vi "Pump Close Selection.vi"(8 "error in (no error)":errorcluster, 11 "Pump Settings In":T1 {"Masterflex"."Pump Number" min=1.0 max=20.0 step=1.0; "Ismatech"."Pump Number" min=1.0 max=20.0 step=1.0; "ASIA Pump C"."channel" min=-1 max=1 step=1}) -> (0 "error out":errorcluster, 1 "Connection Error":bool, 3 "Pump Settings Out":T1 {"Masterflex"."Pump Number" min=1.0 max=20.0 step=1.0; "Ismatech"."Pump Number" min=1.0 max=20.0 step=1.0; "ASIA Pump C"."channel" min=-1 max=1 step=1})   [LabVIEW 2018, in "Pump Module.lvlib" / "Pump Module Engine.lvlib"]
uses:
  Measure Instrument/Pump Module Engine.lvlib
  Measure Instrument/Pump Settings Cluster.ctl
  Measure Instrument/PID 2 Output Enum.ctl
  Masterflex 7550-30/Controls/Settings Cluster.ctl
  Ismatec ISM 831C/Controls/Ismatech Settings Cluster.ctl
  VICI M50 Party Mode/Settings Cluster.ctl
  Tacmina QI/Tacmina QI DAQ Setting.ctl
  KNF Pump/Settings Cluster plus SIMDOS.ctl
  ASIA Pump/Pump Settings.ctl
  FLOM Pump/Settings Cluster.ctl
  SSI PR Class/SSI PR Settings Cluster.ctl
  Ismatec ISM 831C/Ismatec ISM 831C.lvlib
  Masterflex 7550-30/Masterflex 7550-30.lvlib
  VICI M50 Party Mode/VICI M6 M50 Party Mode.lvlib
  Tacmina QI/Tacmina QI.lvlib
  KNF Pump/KNF SIMDOS.lvlib
  ASIA Pump.lvlib
  FLOM Pump/FLOM Pump.lvlib
  SSI PR Class/SSI PR Pump.lvlib
  Pump Module.lvlib
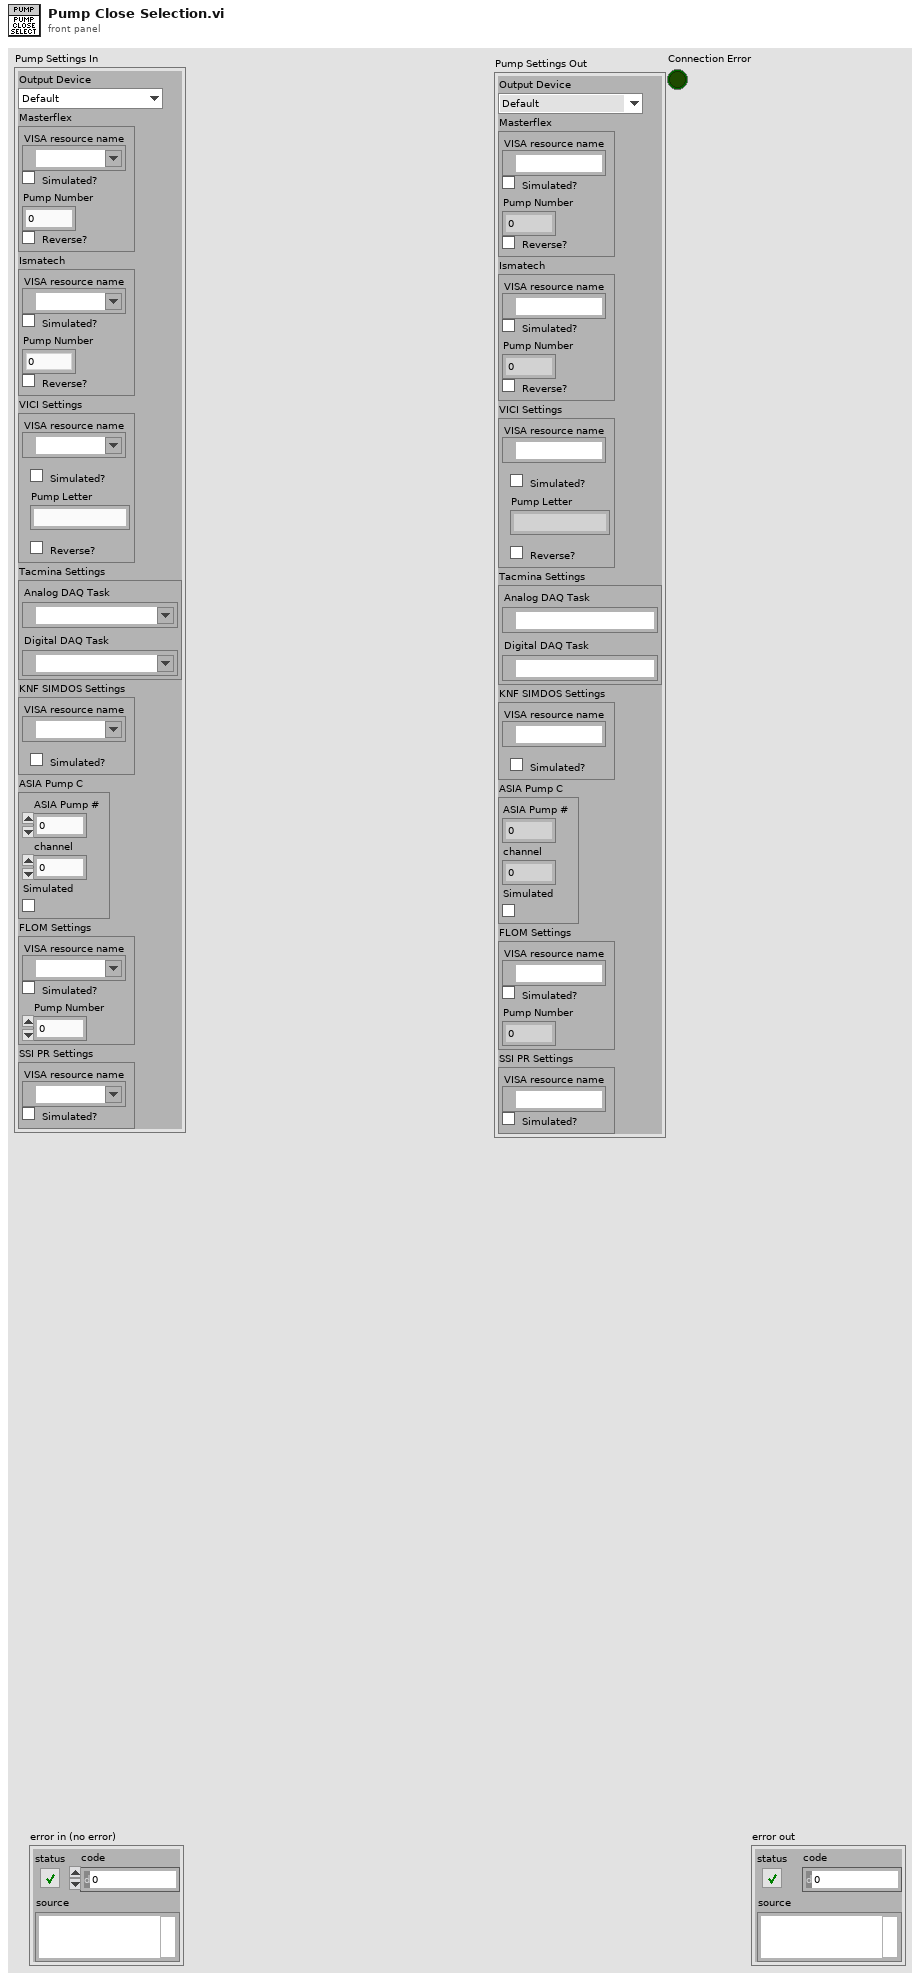
[diagram p1: front panel]
types:
  T1 = typedef "Pump Module.lvlib/Pump Settings Cluster.ctl" = cluster{"Output Device":T2, "Masterflex":T3, "Ismatech":T4, "VICI Settings":T5, "Tacmina Settings":T6, "KNF SIMDOS Settings":T7, "ASIA Pump C":T8, "FLOM Settings":T9, "SSI PR Settings":T10}
  T2 = typedef "PID 2 Output Enum.ctl" = enum16{"Default", "Ismatec ISM 831C", "Masterflex 7550-30", "VICI", "Tacmina QI", "KNF SIMDOS", "ASIA Type C", "FLOM UI-22-11", "SSI PR"}
  T3 = typedef "Masterflex 7550-30.lvlib/Settings Cluster.ctl" = cluster{"VISA resource name":refnum<visa-resource-name>, "Simulated?":bool, "Pump Number":dbl, "Reverse?":bool}
  T4 = typedef "Ismatec ISM 831C.lvlib/Ismatech Settings Cluster.ctl" = cluster{"VISA resource name":refnum<visa-resource-name>, "Simulated?":bool, "Pump Number":dbl, "Reverse?":bool}
  T5 = typedef "VICI M6 M50 Party Mode.lvlib/Settings Cluster.ctl" = cluster{"VISA resource name":refnum<visa-resource-name>, "Simulated?":bool, "Pump Letter":string, "Reverse?":bool}
  T6 = typedef "Tacmina QI.lvlib/Tacmina QI DAQ Setting.ctl" = cluster{"Analog DAQ Task":refnum<k21>, "Digital DAQ Task":refnum<k21>}
  T7 = typedef "KNF SIMDOS.lvlib/Settings Cluster plus SIMDOS.ctl" = cluster{"VISA resource name":refnum<visa-resource-name>, "Simulated?":bool}
  T8 = typedef "ASIA Pump.lvlib/Pump Settings.ctl" = cluster{"ASIA Pump #":i32, "channel":i32, "Simulated":bool}
  T9 = typedef "FLOM Pump.lvlib/Settings Cluster.ctl" = cluster{"VISA resource name":refnum<visa-resource-name>, "Simulated?":bool, "Pump Number":dbl}
  T10 = typedef "SSI PR Pump.lvlib/SSI PR Settings Cluster.ctl" = cluster{"VISA resource name":refnum<visa-resource-name>, "Simulated?":bool}
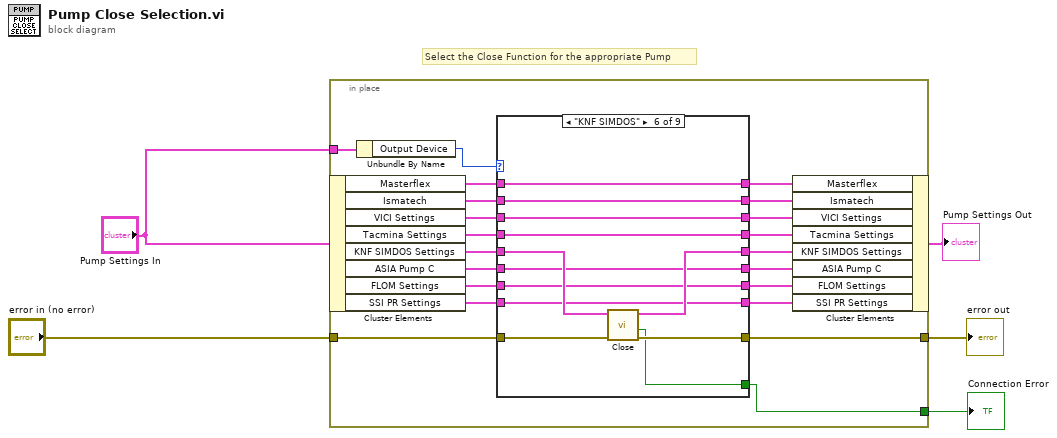
[diagram p0: block diagram]
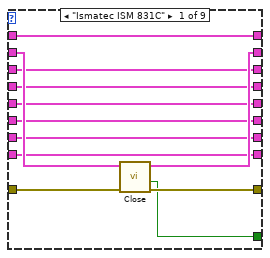
[diagram p2: hidden frame]
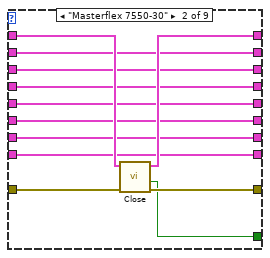
[diagram p3: hidden frame]
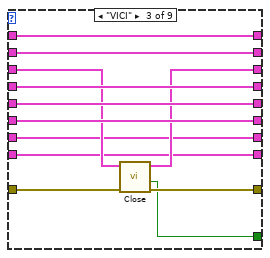
[diagram p4: hidden frame]
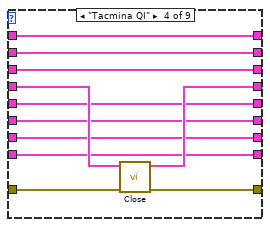
[diagram p5: hidden frame]
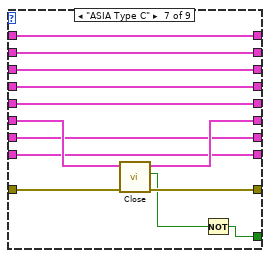
[diagram p7: hidden frame]
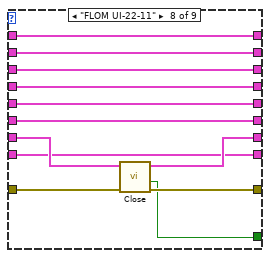
[diagram p8: hidden frame]
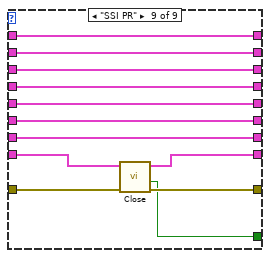
[diagram p9: hidden frame]
diagram:
  # "Select the Close Function for the appropriate Pump"
  n1 = in-place {
    in-place-border: "error in (no error)" -> [w25]
    in-place-border: [w24] -> w4
    in-place-border: "Pump Settings In" -> [w23]
    in-place-border: [w22] -> w3
    n2 = in-place-cluster #1("Pump Settings In") -> ("Masterflex"=w21:T3, "Ismatech"=w20:T4, "VICI Settings"=w19:T5, "Tacmina Settings"=w18:T6, "KNF SIMDOS Settings"=w17:T7, "ASIA Pump C"=w16:T8, "FLOM Settings"=w15:T9, "SSI PR Settings"=w14:T10)
    n3 = Unbundle By Name(w23) -> ("Output Device"=w26:T2)
    n4 = case shown="\"KNF SIMDOS\"" w26 {
      tunnel: w21 -> [w34 w50 w59 w70 w82 w94 w105 w119 w131]
      tunnel: [w34 w49 w59 w70 w82 w94 w105 w119 w131] -> w13
      tunnel: w20 -> [w36 w47 w60 w71 w81 w93 w104 w118 w130]
      tunnel: [w38 w48 w61 w72 w80 w90 w106 w112 w123] -> w24
      tunnel: w25 -> [w37 w46 w62 w73 w80 w91 w107 w113 w124]
      tunnel: [w35 w47 w60 w71 w81 w93 w104 w118 w130] -> w12
      tunnel: [w33 w45 w58 w69 w79 w92 w103 w116 w128] -> w10
      tunnel: w18 -> [w33 w45 w58 w68 w79 w92 w103 w116 w128]
      tunnel: [w32 w44 w57 w67 w78 w89 w102 w115 w127] -> w9
      tunnel: w17 -> [w32 w44 w57 w67 w78 w88 w102 w115 w127]
      tunnel: w16 -> [w31 w43 w56 w66 w77 w87 w101 w114 w126]
      tunnel: [w31 w43 w56 w66 w77 w87 w100 w114 w126] -> w8
      tunnel: [w30 w42 w55 w65 w76 w86 w99 w117 w129] -> w11
      tunnel: w19 -> [w30 w42 w54 w65 w76 w86 w99 w117 w129]
      tunnel: [w29 w41 w53 w64 w75 w85 w98 w110 w125] -> w7
      tunnel: w15 -> [w29 w41 w53 w64 w75 w85 w98 w111 w125]
      tunnel: w14 -> [w28 w40 w52 w63 w74 w84 w97 w109 w121]
      tunnel: [w28 w40 w52 w63 w74 w84 w97 w109 w122] -> w6
      tunnel: [w27 w39 w51 _ _ w83 w96 w108 w120] -> w22
      frame "Ismatec ISM 831C" {
        n5 = call "Close.vi"("error in (no error)"=w37, "Ismatech Settings"=w36) -> ("error out"=w38:errorcluster, "Connection Error"=w27:bool, "Ismatech Settings"=w35:T4)  [unwired: 7 in]
      }
      frame "Masterflex 7550-30" {
        n6 = call "Close.vi"("error in (no error)"=w46, "Masterflex Settings in"=w50) -> ("error out"=w48:errorcluster, "Connection Error"=w39:bool, "Masterflex Settings out"=w49:T3)  [unwired: 7 in]
      }
      frame "VICI" {
        n7 = call "Close.vi"("error in (no error)"=w62, "VICI Settings"=w54) -> ("error out"=w61:errorcluster, "Connection Error"=w51:bool, "VICI Settings"=w55:T5)  [unwired: 7 in]
      }
      frame "Tacmina QI" {
        n8 = call "Close.vi"("error in"=w73, "Tacmina Settings in"=w68) -> ("error out"=w72:errorcluster, "Tacmina Settings out"=w69:T6)  [unwired: 8 in]
      }
      frame "Default", Default {
      }
      frame "KNF SIMDOS" {
        n9 = call "Close.vi"("error in (no error)"=w91, "KNF Settings"=w88) -> ("error out"=w90:errorcluster, "Connection Error"=w83:bool, "KNF Settings"=w89:T7)  [unwired: 7 in]
      }
      frame "ASIA Type C" {
        n10 = call "Close.vi"("error in (no error)"=w107, "ASIA Pump C"=w101) -> ("error out"=w106:errorcluster, "Task Completed"=w95:bool, "ASIA Pump C"=w100:T8)  [unwired: 7 in]
        n11 = Not(x=w95) -> (.not. x?=w96:bool)
      }
      frame "FLOM UI-22-11" {
        n12 = call "Close.vi"("error in (no error)"=w113, "FLOM Settings in"=w111) -> ("error out"=w112:errorcluster, "Connection Error"=w108:bool, "FLOM Settings out"=w110:T9)  [unwired: 7 in]
      }
      frame "SSI PR" {
        n13 = call "Close.vi"("error in (no error)"=w124, "SSI PR Settings In"=w121) -> ("error out"=w123:errorcluster, "Connection Error"=w120:bool, "SSI PR Settings Out"=w122:T10)  [unwired: 7 in]
      }
    }
    n14 = in-place-cluster #1("Masterflex"=w13, "Ismatech"=w12, "VICI Settings"=w11, "Tacmina Settings"=w10, "KNF SIMDOS Settings"=w9, "ASIA Pump C"=w8, "FLOM Settings"=w7, "SSI PR Settings"=w6) -> (→"Pump Settings Out":T1)
  }
  "error out" <- w4
  "Connection Error" <- w3
